vi "Write VISA resource name.vi"(8 "error in (no error)":errorcluster, 10 "VISA resource name":refnum<visa-resource-name>="TCPIP0::192.168.1.69::1852::SOCKET", 11 "Strain Digitizer in":refnum<class "Strain Digitizer.lvclass">) -> (0 "error out":errorcluster, 3 "Strain Digitizer out":refnum<class "Strain Digitizer.lvclass">)   [LabVIEW 2015, in "Strain Digitizer.lvclass"]
uses:
  Strain Digitizer.lvclass
  Strain Digitizer.lvclass/Strain Digitizer.ctl
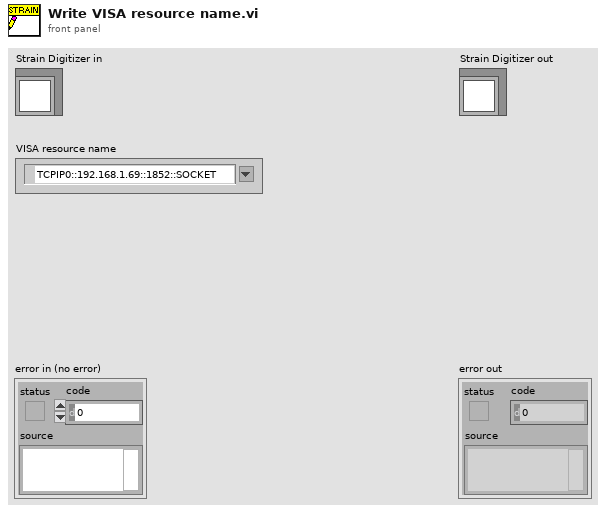
[diagram p1: front panel]
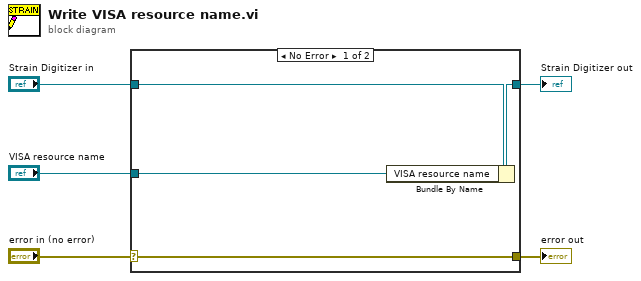
[diagram p0: block diagram]
diagram:
  n1 = case shown="No Error" "error in (no error)" {
    selector: "error in (no error)" -> [w9 w10]
    tunnel: [w9 w10] -> w4
    tunnel: [w7 w11] -> w2
    tunnel: "Strain Digitizer in" -> [w8 w11]
    tunnel: "VISA resource name" -> [w6 _]
    frame No Error {
      n2 = Bundle By Name(cluster=w8, "VISA resource name"=w6) -> (w7:refnum<class "Strain Digitizer.lvclass">)
    }
    frame Error {
    }
  }
  "error out" <- w4
  "Strain Digitizer out" <- w2
